vi "Get Test Name.vi"(8 "error in (no error)":errorcluster) -> (0 "error out":errorcluster, 2 "Test":string)   [LabVIEW 2015]
panel:
  in  "Test":i32(listbox)
  in  "OK Button":bool
  out "Test Sequence":i32(listbox)=-2
  # "Select Test"
  # "Please select the type of\ntest you would like to\nexecute"
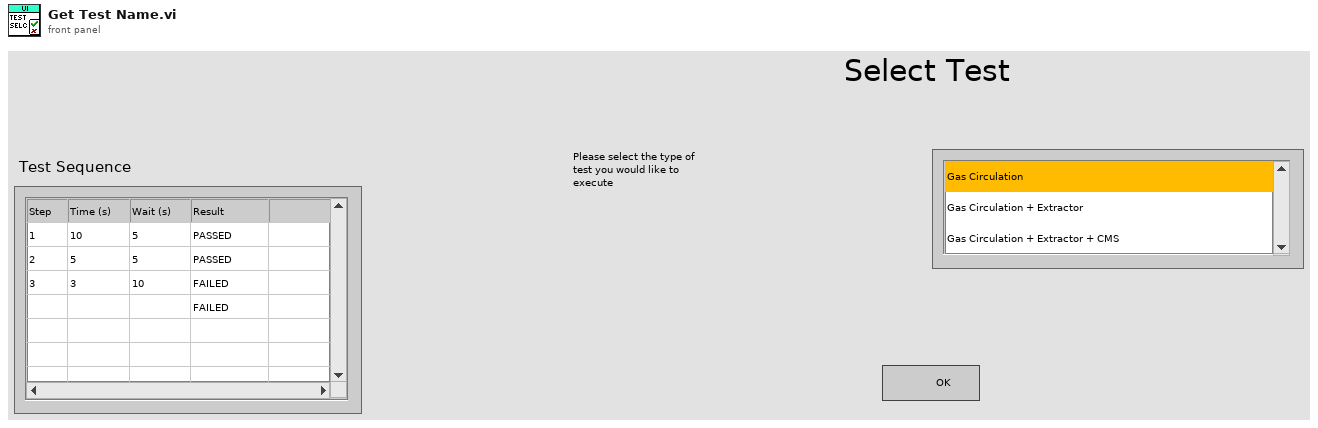
[diagram p1: front panel]
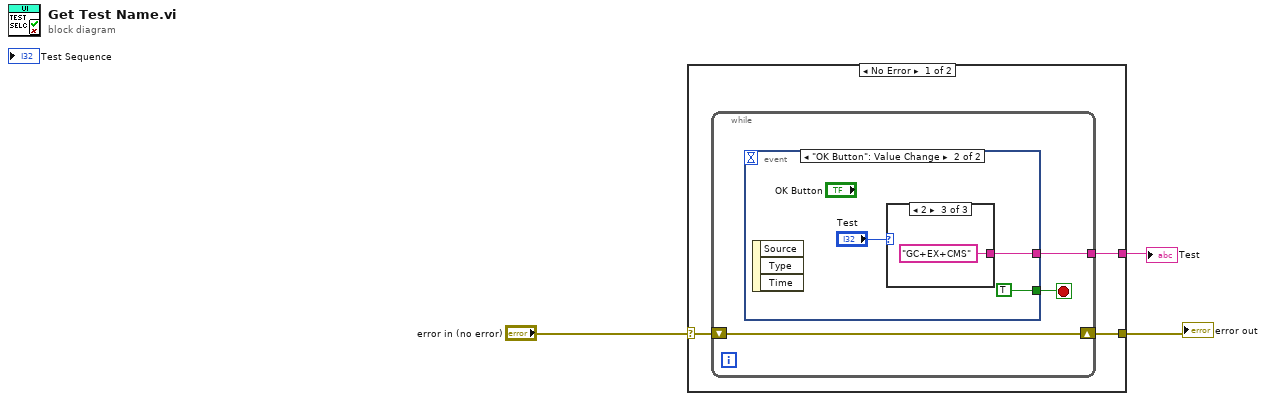
[diagram p0: block diagram]
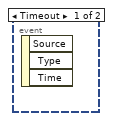
[diagram p2: hidden frame]
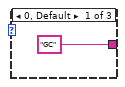
[diagram p3: hidden frame]
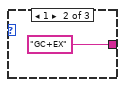
[diagram p4: hidden frame]
diagram:
  n1 = case shown="No Error" "error in (no error)" {
    selector: "error in (no error)" -> [w6 w16]
    tunnel: [w5 w16] -> w3
    tunnel: [w4 _] -> w1
    frame No Error {
      n2 = while {
        shift-right: [w8] -> w5
        shift-left: w6 -> [w8]
        tunnel: [w7] -> w4
        stop <- w9 stop-if-true
        n3 = event shown="[1] \"OK Button\": Value Change" {
          selector: _ -> [_ _]
          dyn-events: _ -> [_ _]
          timeout: _ -> [_ _]
          tunnel: [_ TRUE] -> w9
          tunnel: [_ w10] -> w7
          event Timeout {
            n4 = event-data() -> ()  [unwired: 1 in, 3 out]
          }
          event "OK Button": Value Change {
            n5 = event-data() -> ()  [unwired: 1 in, 3 out]
            n6 = case shown="2" "Test" {
              tunnel: ["GC" "GC+EX" "GC+EX+CMS"] -> w10
              frame 0, Default {
              }
              frame 1 {
              }
              frame 2 {
              }
            }
          }
        }
      }
    }
    frame Error {
    }
  }
  "error out" <- w3
  "Test" <- w1
